vi "UIRef.vi"(8 "error in":errorcluster, 11 "CVT editor node in":refnum<class "CVT editor node.lvclass">) -> (0 "error out":errorcluster, 2 "VI refnum":refnum<vi>, 3 "CVT editor node out":refnum<class "CVT editor node.lvclass">)   [LabVIEW 2013, in "CVT editor node.lvclass"]
uses:
  CVT editor node.lvclass
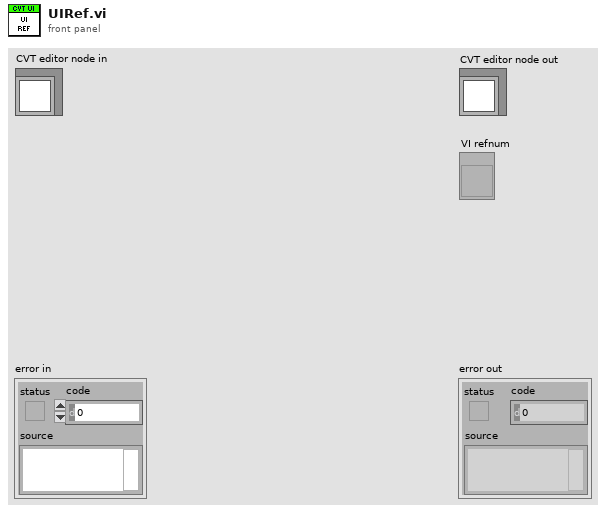
[diagram p1: front panel]
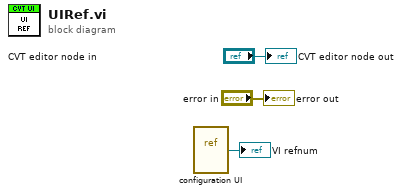
[diagram p0: block diagram]
diagram:
  n1 = vi-ref "configuration UI.vi"() -> (→"VI refnum":refnum<vi>)
  "error out" <- "error in"
  "CVT editor node out" <- "CVT editor node in"
